vi "MS5607-02BA03 Pressure Sensor.vi"() -> ()   [LabVIEW 2014]
doc: "This example demonstrates how to read X, Y, and Z accelerations using the MMA8452 accelerometer."
uses:
  <vilib>/MakerHub/LINX/Public/Utilities/Open Serial.vi
  <vilib>/MakerHub/LINX/LMH-LINX.lvlib
panel:
  out "Waveform Chart":waveform(sgl)[](graph)
  out "Pass CRC?":bool
  out "Press. (mm Hg)":dbl format="%.2g"
  out "Press. (mbar)":dbl format="%#.1f"
  in  "Altitude (ft)":dbl=800.0
  out "Raw Pr (mbar)":dbl
  out "Temp. (C)":dbl format="%.1g"
  in  "I2C Slave Addr.":u8=119 format="%.0x"
  in  "Stop Button":bool
  in  "I2C Channel":u8
  in  "Serial Port":refnum<visa-resource-name>="COM9"
  # "29124 Altimeter Module"
  # "LINX Device Settings"
  # "Outputs"
  # "Pressure  Settings"
  # "Intermediate Results"
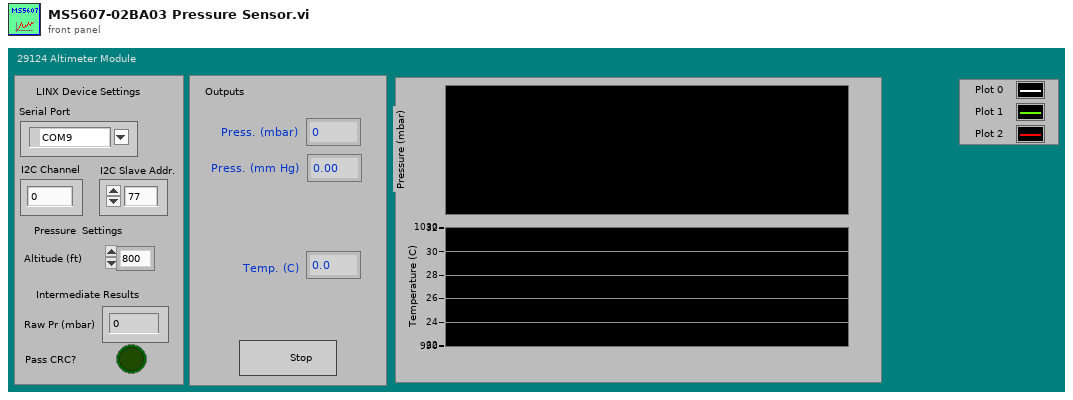
[diagram p1: front panel]
types:
  T1 = typedef "LMH-LINX.lvlib/LINX Ref.ctl" = cluster{"IO":T2, "Interface":T3, "LINX Device Config":T4}
  T2 = typedef "LMH-LINX.lvlib/Platform.ctl" = enum16{"Remote", "Local"}
  T3 = typedef "LMH-LINX.lvlib/Interface.ctl" = enum16{"Serial", "TCP"}
  T4 = typedef "LMH-LINX.lvlib/Device.lvlib/LINX Device Config.ctl" = cluster{"Interface":T3, "COM Port":refnum<visa-resource-name>, "TCP Configuration":T5, "Device Family":u8, "Device ID":u8, "Device Name":string, "TCP Ref":refnum<k5>, "Channels":T6}
  T5 = typedef "LMH-LINX.lvlib/Device.lvlib/TCP Config.ctl" = cluster{"IP Address":string, "Port":u16}
  T6 = typedef "LMH-LINX.lvlib/Channels.ctl" = cluster{"DI":u8[], "DO":u8[], "AI":u8[], "AO":u8[], "PWM":u8[], "QE":u8[], "UART":u8[], "I2C 2":u8[], "SPI":u8[], "CAN":u8[], "Servo":u8[], "AI Ref (V)":dbl, "AI Resolution (Bits)":u8, "AO Ref (V)":dbl, "AO Resolution (Bits)":u8}
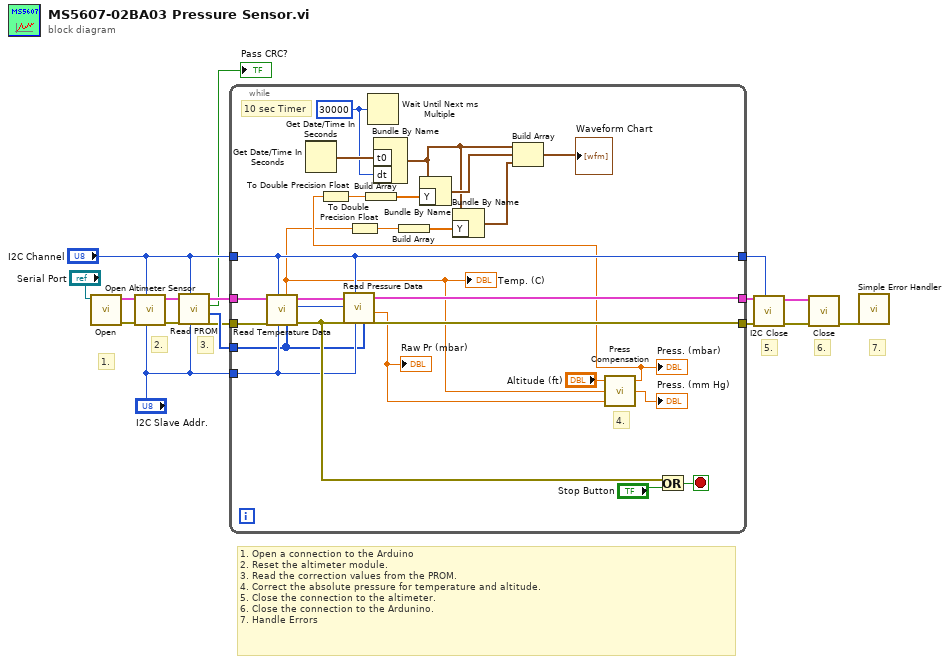
[diagram p0: block diagram]
diagram:
  # "3."
  # "7."
  # "5."
  # "2."
  # "6."
  # "1. Open a connection to the Arduino\n2. Reset the altimeter module.\n3. Read the correction values from the PROM.\n4. Correct the absolute pressure for temperature and altitude.\n5. Close the connection to the altimeter.\n6. Close the connection to the Ardunino.\n7. Handle Errors"
  # "1."
  n1 = call-poly <vilib>:"Open.vi"("Serial Port"="Serial Port") -> ("Error Out"=w16:errorcluster, "LINX Resource"=w15:T1)  [unwired: 8 in, 1 out]
  n2 = call "Open Altimeter Sensor.vi"("I2C Slave Address"="I2C Slave Addr.", "I2C Channel"="I2C Channel", "Error In"=w16, "LINX Ref"=w15) -> ("Error Out"=w3:errorcluster, "LINX Resource"=w4:T1)  [unwired: 6 in]
  n3 = call "Read PROM.vi"("I2C Slave Address"="I2C Slave Addr.", "I2C Channel"="I2C Channel", "Error In"=w3, "LINX Resource in"=w4) -> ("Error Out"=w6:errorcluster, "Correction Values"=w8:u16[], "Pass CRC?"=→"Pass CRC?":bool, "LINX Resource out"=w7:T1)  [unwired: 4 in]
  n4 = while {
    tunnel: "I2C Channel" -> [w36]
    tunnel: "I2C Slave Addr." -> [w35]
    tunnel: [w36] -> w9
    tunnel: w8 -> [w34]
    tunnel: w7 -> [w42]
    tunnel: [w38] -> w12
    tunnel: w6 -> [w41]
    tunnel: [w37] -> w13
    stop <- w43 stop-if-true
    w25 = u32 30000 ("milliseconds to wait")
    # "10 sec Timer"
    # "4."
    n5 = call "Read Temperature Data.vi"("PROM correction Values"=w34, "I2C Slave Address"=w35, "I2C Channel"=w36, "Error In"=w41, "LINX Resource in"=w42) -> ("Error Out"=w40:errorcluster, "dT"=w33:i32, "LINX Resource out"=w39:T1, "Temp"=w20:dbl)  [unwired: 3 in]
    "Temp. (C)" <- w20
    n6 = Get Date/Time In Seconds() -> ()  [unwired: 1 out]
    n7 = Get Date/Time In Seconds() -> (seconds since 1Jan1904=w29:timestamp)
    n8 = call "Read Pressure Data.vi"("PROM correction Values"=w34, "I2C Slave Address"=w35, "I2C Channel"=w36, "Error In"=w40, "dT"=w33, "LINX Resource in"=w39) -> ("Error Out"=w37:errorcluster, "Pr mbar"=w30:dbl, "LINX Resource out"=w38:T1)  [unwired: 3 in]
    "Raw Pr (mbar)" <- w30
    n9 = To Double Precision Float(number=w20) -> (double precision float=w24:dbl)
    n10 = Wait Until Next ms Multiple(millisecond multiple=w25) -> ()  [unwired: 1 out]
    n11 = Bundle By Name("t0"=w29, "dt"=w25) -> (w22:waveform(sgl))  [unwired: 1 in]
    n12 = Build Array(w24) -> (w23:dbl[])
    n13 = Bundle By Name(cluster=w22, "Y"=w23) -> (w19:waveform(sgl))
    n14 = call "Press Compensation.vi"("P abs (mb)"=w30, "Temperature (C)"=w20, "Altitude (ft)"="Altitude (ft)") -> ("Press_Hg"=→"Press. (mm Hg)":dbl, "Press_hPa"=w21:dbl)  [unwired: 1 out]
    "Press. (mbar)" <- w21
    n15 = To Double Precision Float(number=w21) -> (double precision float=w27:dbl)
    n16 = Build Array(w27) -> (w26:dbl[])
    n17 = Bundle By Name(cluster=w22, "Y"=w26) -> (w28:waveform(sgl))
    n18 = Build Array(w22, w28, w19) -> (→"Waveform Chart":waveform(sgl)[])
    n19 = Or(x=w40, y="Stop Button") -> (x .or. y?=w43:bool)
  }
  n20 = call <vilib>:"I2C Close.vi"("I2C Channel (0)"=w9, "Error In"=w13, "LINX Resource"=w12) -> ("Error Out"=w10:errorcluster, "LINX Resource"=w11:T1)  [unwired: 7 in]
  n21 = call <vilib>:"Close.vi"("Error In"=w10, "LINX Resource"=w11) -> ("Error Out"=w14:errorcluster)  [unwired: 9 in]
  n22 = call <vilib>:"Simple Error Handler.vi"("error in (no error)"=w14) -> ()  [unwired: 4 in, 5 out]
